vi "Read Controller Data.vi"(6 "wait for reply (T)":bool=TRUE, 8 "error in":errorcluster, 10 "Temp Units":T1, 11 "Module ID":i32=-1) -> (0 "error out":errorcluster, 1 "timed out?":bool, 2 "Temp Setpoint":T2, 3 "Chamber Temp":T2, 5 "Chamber Output":dbl)   [LabVIEW 2024, in "Thermal Chamber.lvlib"]
doc: "_____\nCreated using DQMH Event Scripter 6.1.0.128."
uses:
  Thermal Chamber.lvlib
  Class Libraries/Process Controller/Controls/Temp Data--Cluster.ctl
  Class Libraries/Process Controller/Controls/Temperature Units--Enum.ctl
  Read Controller Data Argument--cluster.ctl
  Read Controller Data (Reply Payload)--cluster.ctl
  Class Libraries/Process Controller/_Thermal Process Controller.lvclass
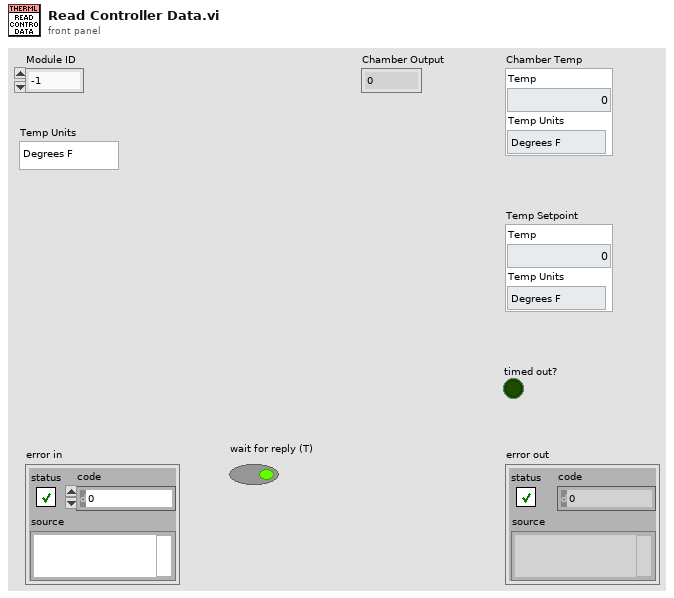
[diagram p1: front panel]
types:
  T1 = typedef "_Thermal Process Controller.lvclass/Temperature Units--Enum.ctl" = enum16{"Degrees F", "Degrees C", "Degrees K"}
  T2 = typedef "_Thermal Process Controller.lvclass/Temp Data--Cluster.ctl" = cluster{"Temp":dbl, "Temp Units":T1}
  T3 = typedef "Thermal Chamber.lvlib/Read Controller Data Argument--cluster.ctl" = cluster{"Module ID":i32, "Temp Units":T1, "Wait Notifier":refnum<notifier>, "wait for reply":bool}
  T4 = typedef "Thermal Chamber.lvlib/Request Events--cluster.ctl" = cluster{"Stop Module":refnum<user-event>, "Show Panel":refnum<user-event>, "Hide Panel":refnum<user-event>, "Show Diagram":refnum<user-event>, "Get Module Execution Status":refnum<user-event>, "Initialize":refnum<user-event>, "Shutdown":refnum<user-event>, "Set Temp Setpoint":refnum<user-event>, "Set Temp Ramp Rate":refnum<user-event>, "Set Temp Control State":refnum<user-event>, "Get Temp Feedback":refnum<user-event>, "Read Controller Data":refnum<user-event>}
  T5 = typedef "Thermal Chamber.lvlib/Read Controller Data (Reply Payload)--cluster.ctl" = cluster{"Chamber Temp":T2, "Temp Setpoint":T2, "Chamber Output":dbl, "error":errorcluster, "Module ID":i32}
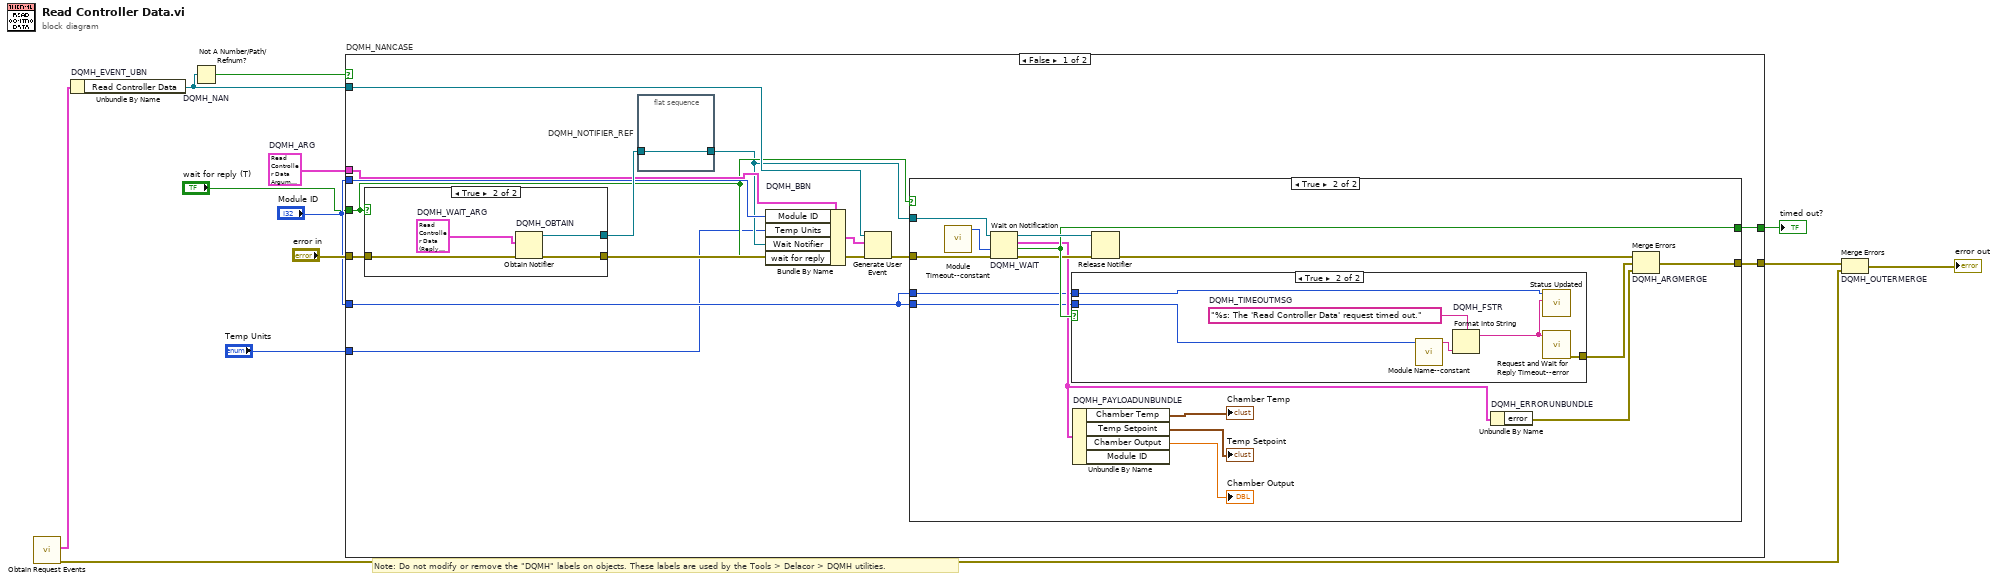
[diagram p0: block diagram]
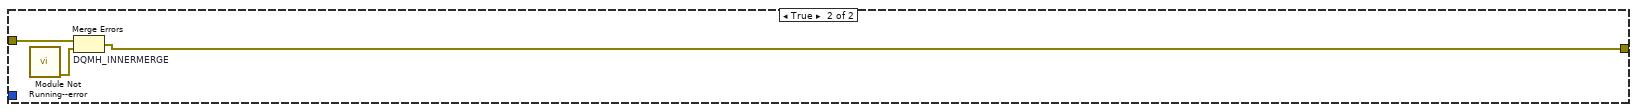
[diagram p5: hidden frame]
diagram:
  w6 = T3 {"Module ID"=-1, "Temp Units"=enum."Degrees F", "Wait Notifier"=refnum, "wait for reply"=FALSE}  # DQMH_ARG
  # "Note: Do not modify or remove the \"DQMH\" labels on objects. These labels are used by the Tools > Delacor > DQMH utilities."
  n1 = call "Obtain Request Events.vi"() -> ("error out"=w3:errorcluster, "Thermal Chamber Request Events"=w2:T4)  [unwired: 10 in]
  n2 = Unbundle By Name "DQMH_EVENT_UBN"(w2) -> ("Read Controller Data"=w10:refnum<user-event>)
  n3 = Not A Number/Path/Refnum? "DQMH_NAN"(number/path/refnum=w10) -> (NaN/Path/Refnum?=w9:bool)
  n4 = case "DQMH_NANCASE" shown="False" w9 {
    tunnel: "error in" -> [w26 w58]
    tunnel: w10 -> [w24 _]
    tunnel: [w21 w57] -> w7
    tunnel: [w22 _] -> w8
    tunnel: w6 -> [w18 _]
    tunnel: "Module ID" -> [w17 _]
    tunnel: "Module ID" -> [w16 _]
    tunnel: "wait for reply (T)" -> [w15 _]
    tunnel: "Temp Units" -> [w13 _]
    frame False {
      n5 = case shown="True" w15 {
        tunnel: w26 -> [w51 w55]
        tunnel: [w51 w54] -> w23
        tunnel: [_ w52] -> w19
        frame False {
        }
        frame True {
          w53 = T5 {"Chamber Temp"={"Temp"=0.0, "Temp Units"=enum."Degrees F"}, "Temp Setpoint"={"Temp"=0.0, "Temp Units"=enum."Degrees F"}, "Chamber Output"=0.0, "error"={"status"=FALSE, "code"=0, "source"=""}, "Module ID"=0}  # DQMH_WAIT_ARG
          n6 = Obtain Notifier "DQMH_OBTAIN"(notification data type=w53, error in (no error)=w55) -> (notifier out=w52:refnum<notifier>, error out=w54:errorcluster)  [unwired: 2 in, 1 out]
        }
      }
      n7 = flat-sequence "DQMH_NOTIFIER_REF" {
        tunnel: w19 -> [w27]
        tunnel: [w27] -> w14
        frame #0 {
        }
      }
      n8 = Bundle By Name "DQMH_BBN"(cluster=w18, "Module ID"=w17, "Temp Units"=w13, "Wait Notifier"=w14, "wait for reply"=w15) -> (w20:T3)
      n9 = Generate User Event(user event=w24, event data cluster=w20, error in=w23) -> (error out=w25:errorcluster)  [unwired: 1 in, 1 out]
      n10 = case shown="True" w15 {
        tunnel: w25 -> [w28 w44]
        tunnel: w14 -> [_ w43]
        tunnel: [_ w41] -> w22
        tunnel: [w28 w40] -> w21
        tunnel: w16 -> [_ w30]
        tunnel: w16 -> [_ w29]
        frame False {
        }
        frame True {
          n11 = call "Module Timeout--constant.vi"() -> ("Module Timeout"=w34:i32)  [unwired: 11 in]
          n12 = Wait on Notification "DQMH_WAIT"(notifier=w43, timeout in ms (-1)=w34, error in (no error)=w44) -> (notifier out=w42:refnum<notifier>, notification=w35:T5, timed out?=w41:bool, error out=w39:errorcluster)  [unwired: 1 in]
          n13 = case shown="True" w41 {
            tunnel: [_ w48] -> w36
            tunnel: w30 -> [_ w46]
            tunnel: w29 -> [_ w45]
            frame False {
            }
            frame True {
              w50 = "%s: The 'Read Controller Data' request timed out."  # DQMH_TIMEOUTMSG
              n14 = call "Module Name--constant.vi"("Module ID"=w45) -> ("Module Name"=w47:string)  [unwired: 10 in]
              n15 = Format Into String "DQMH_FSTR"(format string=w50, w47) -> (resulting string=w49:string)  [unwired: 2 in, 1 out]
              n16 = call "Status Updated.vi"("Status"=w49, "Module ID"=w46) -> ()  [unwired: 9 in, 1 out]
              n17 = call "Request and Wait for Reply Timeout--error.vi"("Error Message"=w49) -> ("error out"=w48:errorcluster)  [unwired: 10 in]
            }
          }
          n18 = Unbundle By Name "DQMH_PAYLOADUNBUNDLE"(w35) -> ("Chamber Temp"=→"Chamber Temp":T2, "Temp Setpoint"=→"Temp Setpoint":T2, "Chamber Output"=→"Chamber Output":dbl)  [unwired: 1 out]
          n19 = Release Notifier(notifier=w42, error in (no error)=w39) -> (error out=w38:errorcluster)  [unwired: 1 in, 2 out]
          n20 = Unbundle By Name "DQMH_ERRORUNBUNDLE"(w35) -> ("error"=w37:errorcluster)
          n21 = Merge Errors "DQMH_ARGMERGE"(w38, w36, w37) -> (w40:errorcluster)
        }
      }
    }
    frame True {
      n22 = call "Module Not Running--error.vi"() -> ("error out"=w56:errorcluster)  [unwired: 11 in]
      n23 = Merge Errors "DQMH_INNERMERGE"(w58, w56) -> (w57:errorcluster)
    }
  }
  "timed out?" <- w8
  n24 = Merge Errors "DQMH_OUTERMERGE"(w7, w3) -> (→"error out":errorcluster)
